vi "Save Reaction Rover Data to Experiment File.vi"(8 "error in (no error)":errorcluster, 11 "Reaction Rover Data":T1={"Visible Hardware VI"="", "Current Message"={"Source"="", "Destination"="", "Time Stamp"=timestamp(0 s since 1904-01-01), "Command"="", "Data"=variant(string "")}, "Message History"=[], "Hardware"={"Process Cache"=refnum, "Plugins"=[{"Plugin Name"="", "Controller Type"=enum."Invalid", "Control Panel Path"=path "", "Plugin Type"=enum."Optimizer"}, {"Plugin Name"="", "Controller Type"=enum."Invalid", "Control Panel Path"=path "", "Plugin Type"=enum."Optimizer"}, {"Plugin Name"="", "Controller Type"=enum."Invalid", "Control Panel Path"=path "", "Plugin Type"=enum."Optimizer"}, {"Plugin Name"="", "Controller Type"=enum."Invalid", "Control Panel Path"=path "", "Plugin Type"=enum."Optimizer"}]}, "Optimizers"={"Process Cache"=refnum, "Plugins"=[{"Plugin Name"="", "Controller Type"=enum."Invalid", "Control Panel Path"=path "", "Plugin Type"=enum."Optimizer"}, {"Plugin Name"="", "Controller Type"=enum."Invalid", "Control Panel Path"=path "", "Plugin Type"=enum."Optimizer"}, {"Plugin Name"="", "Controller Type"=enum."Invalid", "Control Panel Path"=path "", "Plugin Type"=enum."Optimizer"}], "First parameteres?"=FALSE, "New Parameters"={"Time Stamp"=timestamp(0 s since 1904-01-01), "Names"=[], "Values"=[]}}, "Parameter to Hardware Map"=refnum, "Analyzers"={"Process Cache"=refnum, "Plugins"=[{"Plugin Name"="", "Controller Type"=enum."Invalid", "Control Panel Path"=path "", "Plugin Type"=enum."Optimizer"}, {"Plugin Name"="", "Controller Type"=enum."Invalid", "Control Panel Path"=path "", "Plugin Type"=enum."Optimizer"}, {"Plugin Name"="", "Controller Type"=enum."Invalid", "Control Panel Path"=path "", "Plugin Type"=enum."Optimizer"}, {"Plugin Name"="", "Controller Type"=enum."Invalid", "Control Panel Path"=path "", "Plugin Type"=enum."Optimizer"}]}, "Log Directory"=path "", "Auto Pass Parameters"=FALSE, "Experiment"={"Name"="", "File Path"=path "", "File Extension"="", "File Cluster"={"Hardware List"=[], "Optimizer List"=[], "Analyzer List"=[], "Parameter to Hardware Map"=[]}}, "Main VI Queue"=refnum, "Process Queue References"=[], "Message Queue"=refnum}) -> (0 "error out":errorcluster, 2 "cancelled":bool, 3 "Reaction Rover Data out":T1={"Visible Hardware VI"="", "Current Message"={"Source"="", "Destination"="", "Time Stamp"=timestamp(0 s since 1904-01-01), "Command"="", "Data"=variant(string "")}, "Message History"=[], "Hardware"={"Process Cache"=refnum, "Plugins"=[{"Plugin Name"="", "Controller Type"=enum."Invalid", "Control Panel Path"=path "", "Plugin Type"=enum."Optimizer"}, {"Plugin Name"="", "Controller Type"=enum."Invalid", "Control Panel Path"=path "", "Plugin Type"=enum."Optimizer"}, {"Plugin Name"="", "Controller Type"=enum."Invalid", "Control Panel Path"=path "", "Plugin Type"=enum."Optimizer"}, {"Plugin Name"="", "Controller Type"=enum."Invalid", "Control Panel Path"=path "", "Plugin Type"=enum."Optimizer"}]}, "Optimizers"={"Process Cache"=refnum, "Plugins"=[{"Plugin Name"="", "Controller Type"=enum."Invalid", "Control Panel Path"=path "", "Plugin Type"=enum."Optimizer"}, {"Plugin Name"="", "Controller Type"=enum."Invalid", "Control Panel Path"=path "", "Plugin Type"=enum."Optimizer"}, {"Plugin Name"="", "Controller Type"=enum."Invalid", "Control Panel Path"=path "", "Plugin Type"=enum."Optimizer"}], "First parameteres?"=FALSE, "New Parameters"={"Time Stamp"=timestamp(0 s since 1904-01-01), "Names"=[], "Values"=[]}}, "Parameter to Hardware Map"=refnum, "Analyzers"={"Process Cache"=refnum, "Plugins"=[{"Plugin Name"="", "Controller Type"=enum."Invalid", "Control Panel Path"=path "", "Plugin Type"=enum."Optimizer"}, {"Plugin Name"="", "Controller Type"=enum."Invalid", "Control Panel Path"=path "", "Plugin Type"=enum."Optimizer"}, {"Plugin Name"="", "Controller Type"=enum."Invalid", "Control Panel Path"=path "", "Plugin Type"=enum."Optimizer"}, {"Plugin Name"="", "Controller Type"=enum."Invalid", "Control Panel Path"=path "", "Plugin Type"=enum."Optimizer"}]}, "Log Directory"=path "", "Auto Pass Parameters"=FALSE, "Experiment"={"Name"="", "File Path"=path "", "File Extension"="", "File Cluster"={"Hardware List"=[], "Optimizer List"=[], "Analyzer List"=[], "Parameter to Hardware Map"=[]}}, "Main VI Queue"=refnum, "Process Queue References"=[], "Message Queue"=refnum})   [LabVIEW 2020, in "RxnRover.lvlib"]
uses:
  RxnRover.lvlib
  Type Definitions/Data.ctl
  Plugin Servers/Controller Array/Controller Array.lvclass
  Plugin Servers/Parameter to Hardware Map/Parameter to Hardware Map.lvclass
  <userlib>/RxnRover/DynamicReentrant/src/Type Defs/Message.ctl
  Plugin Manager/Plugin Details.ctl
  Plugin Servers/Controller/Controller Type.ctl
  Plugin Manager/Plugin Types.ctl
  Type Definitions/New Parameters.ctl
  Experiment/Experiment File/Experiment File Cluster.ctl
  Plugin Servers/Controller/Minimal Controller Cluster.ctl
  Plugin Servers/Parameter to Hardware Map/Minimal Map.ctl
  Plugin Servers/Parameter to Hardware Map/Minimal Pair Cluster.ctl
  User Preferences/User Preferences File.lvclass
  Experiment/Experiment File/Experiment File.lvlib
  Experiment/Experiment Manager/Experiment Manager.lvlib
  <userlib>/RxnRover/DynamicReentrant/Dynamic Reentrant.lvlib
  Plugin Servers/Controller/Generic Plugin.lvclass
  Plugin Manager/Plugin Manager.lvlib
panel:
  # "Note: Rxn Rover data control and indicator are hidden!"
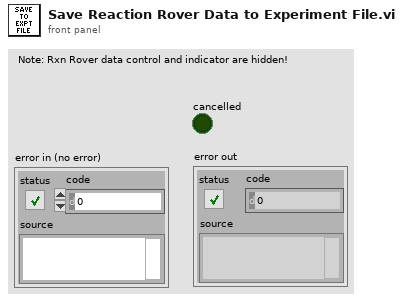
[diagram p1: front panel]
types:
  T1 = typedef "RxnRover.lvlib/Data.ctl" = cluster{"Visible Hardware VI":string, "Current Message":T2, "Message History":string[][], "Hardware":cluster{"Process Cache":refnum<class "Controller Array.lvclass">, "Plugins":T3[]}, "Optimizers":cluster{"Process Cache":refnum<class "Controller Array.lvclass">, "Plugins":T3[], "First parameteres?":bool, "New Parameters":T6}, "Parameter to Hardware Map":refnum<class "Parameter to Hardware Map.lvclass">, "Analyzers":cluster{"Process Cache":refnum<class "Controller Array.lvclass">, "Plugins":T3[]}, "Log Directory":path, "Auto Pass Parameters":bool, "Experiment":cluster{"Name":string, "File Path":path, "File Extension":string, "File Cluster":T7}, "Main VI Queue":refnum<queue>, "Process Queue References":refnum<queue>[], "Message Queue":refnum<queue>}
  T2 = typedef "Dynamic Reentrant.lvlib/Message.ctl" = cluster{"Source":string, "Destination":string, "Time Stamp":timestamp, "Command":string, "Data":variant}
  T3 = typedef "RxnRover.lvlib/Plugin Manager.lvlib/Plugin Details.ctl" = cluster{"Plugin Name":string, "Controller Type":T4, "Control Panel Path":path, "Plugin Type":T5}
  T4 = typedef "RxnRover.lvlib/Generic Plugin.lvclass/Controller Type.ctl" = enum16{"Invalid", "Temperature Controller", "Pump Controller", "Syringe Pump", "Generic Optimizer", "LC Parser"}
  T5 = typedef "RxnRover.lvlib/Plugin Manager.lvlib/Plugin Types.ctl" = enum16{"Invalid", "Optimizer", "Analyzer", "Hardware"}
  T6 = typedef "RxnRover.lvlib/New Parameters.ctl" = cluster{"Time Stamp":timestamp, "Names":string[], "Values":variant[]}
  T7 = typedef "RxnRover.lvlib/Experiment File.lvlib/Experiment File Cluster.ctl" = cluster{"Hardware List":T8[], "Optimizer List":T8[], "Analyzer List":T8[], "Parameter to Hardware Map":T9}
  T8 = typedef "RxnRover.lvlib/Generic Plugin.lvclass/Minimal Controller Cluster.ctl" = cluster{"Name":string, "Controller Type":string, "Control Panel Path":string, "Resource":string}
  T9 = typedef "RxnRover.lvlib/Parameter to Hardware Map.lvclass/Minimal Map.ctl" = T10[]
  T10 = typedef "RxnRover.lvlib/Parameter to Hardware Map.lvclass/Minimal Pair Cluster.ctl" = cluster{"key":string, "values":T8[]}
  T11 = typedef "RxnRover.lvlib/Generic Plugin.lvclass/Minimal Controller Cluster Array.ctl" = T8[]
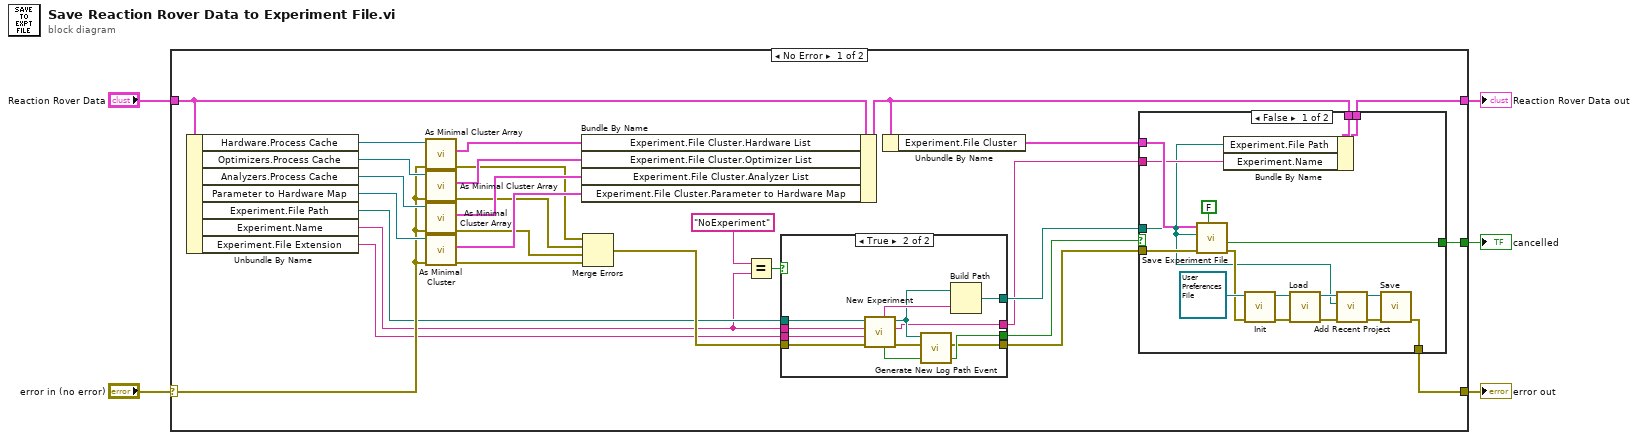
[diagram p0: block diagram]
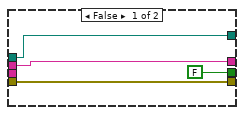
[diagram p2: hidden frame]
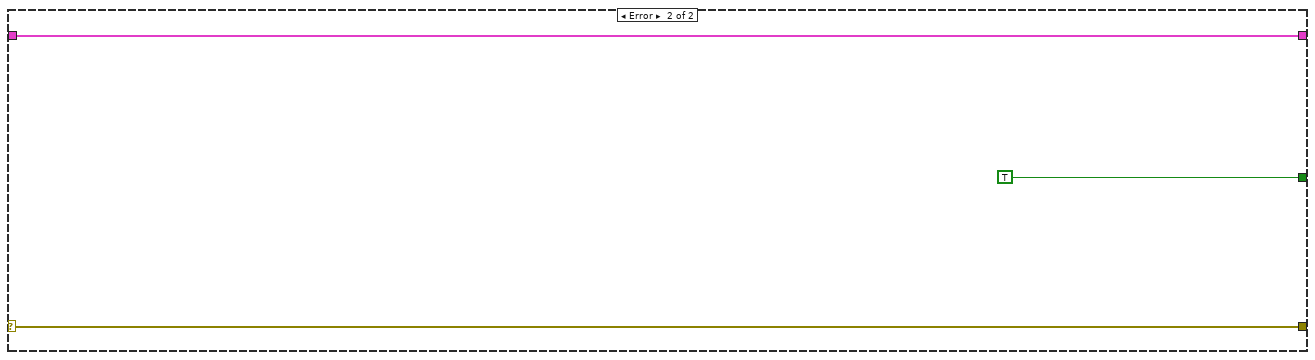
[diagram p4: hidden frame]
diagram:
  n1 = case shown="No Error" "error in (no error)" {
    selector: "error in (no error)" -> [w26 w72]
    tunnel: [w9 w72] -> w4
    tunnel: "Reaction Rover Data" -> [w34 w71]
    tunnel: [w12 w71] -> w2
    tunnel: [w18 TRUE ("cancelled")] -> w1
    frame No Error {
      n2 = Unbundle By Name(w34) -> ("Hardware.Process Cache"=w33:refnum<class "Controller Array.lvclass">, "Optimizers.Process Cache"=w32:refnum<class "Controller Array.lvclass">, "Analyzers.Process Cache"=w31:refnum<class "Controller Array.lvclass">, "Parameter to Hardware Map"=w27:refnum<class "Parameter to Hardware Map.lvclass">, "Experiment.File Path"=w8:path, "Experiment.Name"=w7:string, "Experiment.File Extension"=w11:string)
      n3 = call "As Minimal Cluster Array.vi"("error in (no error)"=w26, "Controller Array in"=w33) -> ("error out"=w24:errorcluster, "Controller Array"=w30:T11)  [unwired: 7 in, 1 out]
      n4 = call "As Minimal Cluster Array.vi"("error in (no error)"=w26, "Controller Array in"=w32) -> ("error out"=w23:errorcluster, "Controller Array"=w29:T11)  [unwired: 7 in, 1 out]
      n5 = call "As Minimal Cluster Array.vi"("error in (no error)"=w26, "Controller Array in"=w31) -> ("error out"=w22:errorcluster, "Controller Array"=w28:T11)  [unwired: 7 in, 1 out]
      n6 = call "As Minimal Cluster.vi"("error in (no error)"=w26, "Parameter to Hardware Map in"=w27) -> ("error out"=w21:errorcluster, "Minimal Parameter to Hardware Map out"=w25:T9)  [unwired: 7 in, 1 out]
      n7 = Bundle By Name(cluster=w34, "Experiment.File Cluster.Hardware List"=w30, "Experiment.File Cluster.Optimizer List"=w29, "Experiment.File Cluster.Analyzer List"=w28, "Experiment.File Cluster.Parameter to Hardware Map"=w25) -> (w13:T1)
      n8 = Merge Errors(w24, w23, w22, w21) -> (w20:errorcluster)
      n9 = Equal?(x="NoExperiment", y=w7) -> (x = y?=w15:bool)
      n10 = case shown="True" w15 {
        tunnel: w20 -> [w38 w45]
        tunnel: [w38 w46] -> w17
        tunnel: [FALSE ("cancelled") w48] -> w16
        tunnel: w8 -> [w35 w44]
        tunnel: [w35 w47] -> w14
        tunnel: w7 -> [w36 w43]
        tunnel: w11 -> [_ w42]
        tunnel: [w36 w39] -> w10
        frame False {
        }
        frame True {
          n11 = call "New Experiment.vi"("error in (no error)"=w45, "Experiment File Extension"=w42, "Experiment Name in"=w43, "Experiment Location in"=w44) -> ("error out"=w49:errorcluster, "Experiment Name out"=w39:string, "Experiment Location out"=w40:path, "cancelled"=w48:bool, "Experiment filename out"=w41:string)  [unwired: 2 in, 1 out]
          n12 = call "Generate New Log Path Event.vi"("error in (no error)"=w49, "New Log Path"=w40) -> ("error out"=w46:errorcluster)  [unwired: 9 in]
          n13 = Build Path(base path=w40, name or relative path=w41) -> (appended path=w47:path)
        }
      }
      n14 = Unbundle By Name(w13) -> ("Experiment.File Cluster"=w19:T7)
      n15 = case shown="False" w16 {
        selector: w16 -> [_ w69]
        tunnel: w19 -> [w66 _]
        tunnel: [w65 w69] -> w18
        tunnel: w14 -> [w50 _]
        tunnel: w17 -> [w63 w67]
        tunnel: w13 -> [w62 w68]
        tunnel: [w61 w68] -> w12
        tunnel: w10 -> [w60 _]
        tunnel: [w51 w67] -> w9
        frame False {
          n16 = call "Save Experiment File.vi"("Confirm Replace File? (T)"=FALSE, "error in (no error)"=w63, "Experiment File Full Path"=w50, "Experiment File Cluster"=w66) -> ("error out"=w52:errorcluster, "cancelled"=w65:bool)  [unwired: 4 in, 2 out]
          n17 = Bundle By Name(cluster=w62, "Experiment.File Path"=w50, "Experiment.Name"=w60) -> (w61:T1)
          n18 = call "Init.vi"("error in (no error)"=w52, "UserPreferencesFileManager in"=refnum<class "User Preferences File.lvclass"> refnum ("User Preferences File.lvclass")) -> ("error out"=w57:errorcluster, "UserPreferencesFileManager out"=w54:refnum<class "User Preferences File.lvclass">)  [unwired: 8 in]
          n19 = call "Load.vi"("error in (no error)"=w57, "User Preferences File in"=w54) -> ("error out"=w55:errorcluster, "User Preferences File out"=w56:refnum<class "User Preferences File.lvclass">)  [unwired: 8 in]
          n20 = call "Add Recent Project.vi"("error in (no error)"=w55, "New Recent Experiment path"=w50, "User Preferences File in"=w56) -> ("error out"=w58:errorcluster, "User Preferences File out"=w59:refnum<class "User Preferences File.lvclass">)  [unwired: 7 in]
          n21 = call "Save.vi"("error in (no error)"=w58, "User Preferences File in"=w59) -> ("error out"=w51:errorcluster)  [unwired: 8 in, 1 out]
        }
        frame True {
        }
      }
    }
    frame Error {
    }
  }
  "error out" <- w4
  "Reaction Rover Data out" <- w2
  "cancelled" <- w1
